vi "EGE.vi"(0 "System no.":i32=1 min=1 max=4 step=1, 2 "Axes to command":string[](array[string]), 3 "Electronic gearing mode":bool[](array[boolean]), 5 "error in":errorcluster, 6 "Without axis ID?":bool) -> (19 "error out":errorcluster)   [LabVIEW 2020]
doc: "Sets electronic gearing mode for given axes. If Without axis ID is TRUE, then Axes to command is ignored and first field of Electronic gearing mode array is used.\n\nC-843: Without axis ID = FALSE. This command can only be issued to a slave axis. The master-slave assignments are set with MAS.vi. Use MAS?.vi to get the current master axis, i.e. the one to be commanded with MOV.vi.\n\nC-848: Without axis ID = FALSE. This command can only be issued to a slave axis. The master-slave assignments are hardware-dependent. Use MAS?.vi to get the related master axis, i.e. the one to be commanded with MOV.vi.\n\nC-880: Without axis ID = FALSE. This command can only be issued to a slave axis. The master-slave assignments are hardware-dependent. Use MAS?.vi to get the related master axis, i.e. the one to be commanded with MOV.vi."
panel:
  # "Sets electronic gearing mode for given axes. If \"Without axis ID\" is \nTRUE, then \"Axes to command\" is ignored and first field of \"Electronic \ngearing mode\" array is used for electronic gearing mode command."
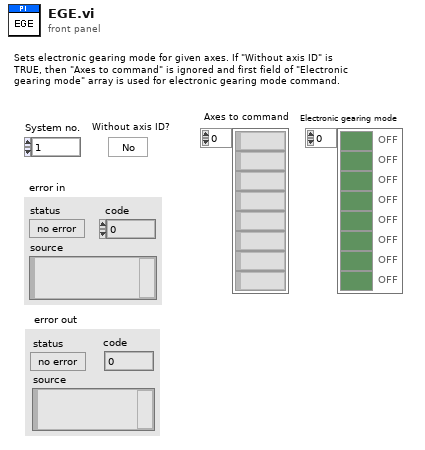
[diagram p1: front panel]
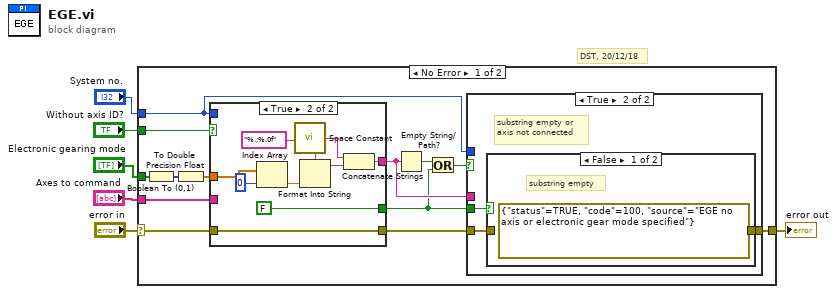
[diagram p0: block diagram]
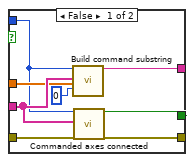
[diagram p2: hidden frame]
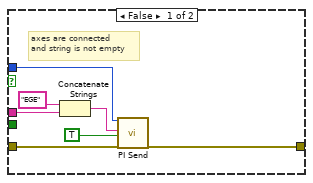
[diagram p3: hidden frame]
diagram:
  # "DST, 20/12/18"
  n1 = case shown="No Error" "error in" {
    selector: "error in" -> [w7 w49]
    tunnel: [w19 w49] -> w6
    tunnel: "System no." -> [w11 _]
    tunnel: "Axes to command" -> [w17 _]
    tunnel: "Electronic gearing mode" -> [w15 _]
    tunnel: "Without axis ID?" -> [w12 _]
    frame No Error {
      n2 = Boolean To (0,1)(Boolean=w15) -> (0, 1=w14:i16[])
      n3 = To Double Precision Float(number=w14) -> (double precision float=w13:dbl[])
      n4 = case shown="True" w12 {
        tunnel: [w27 w31] -> w10
        tunnel: w7 -> [w26 w36]
        tunnel: [w25 w36] -> w18
        tunnel: w17 -> [w24 _]
        tunnel: [w23 FALSE] -> w9
        tunnel: w13 -> [w21 w33]
        tunnel: w11 -> [w20 _]
        frame False {
          n5 = call "Build command substring.vi"("System no."=w20, "Affected axes"=w24, "Parameters"=w21, "No. of digits"=i16 0 ("No.of digits")) -> ("Command substring"=w27:string)  [unwired: 3 in, 12 out]
          n6 = call "Commanded axes connected.vi"("System no."=w20, "Commanded axes"=w24, "error in"=w26) -> ("Controller error"=w23:bool, "error out"=w25:errorcluster)  [unwired: 1 in, 14 out]
        }
        frame True {
          n7 = Index Array(array=w33, index=0 ("Index")) -> (element=w32:dbl)
          n8 = call <vilib>:"Space Constant.vi"() -> ("String"=w29:string)
          n9 = Format Into String(format string="%.;%.0f" ("Format String"), w32) -> (resulting string=w30:string)  [unwired: 2 in, 1 out]
          n10 = Concatenate Strings(w29, w30) -> (w31:string)
        }
      }
      n11 = Empty String/Path?(string/path=w10) -> (empty?=w8:bool)
      n12 = Or(x=w8, y=w9) -> (x .or. y?=w16:bool)
      n13 = case shown="True" w16 {
        tunnel: w10 -> [w42 _]
        tunnel: [w38 w46] -> w19
        tunnel: w18 -> [w39 w44]
        tunnel: w9 -> [_ w45]
        tunnel: w11 -> [w37 _]
        frame False {
          # "axes are connected \nand string is not empty"
          n14 = Concatenate Strings("EGE", w42) -> (w40:string)
          n15 = call "PI Send.vi"("System no."=w37, "String to send"=w40, "Attach termination char.?"=TRUE ("Attach Linefeed?"), "error in"=w39) -> ("error out"=w38:errorcluster)  [unwired: 2 in, 13 out]
        }
        frame True {
          # "substring empty or\naxis not connected"
          n16 = case shown="False" w45 {
            tunnel: [errorcluster {"status"=TRUE, "code"=100, "source"="EGE no axis or electronic gear mode specified"} ("error out") w48] -> w46
            tunnel: w44 -> [_ w48]
            frame False {
              # "substring empty"
            }
            frame True {
              # "commanded axis\nnot connected"
            }
          }
        }
      }
    }
    frame Error {
    }
  }
  "error out" <- w6
